vi "Right Click Menu Selected.vi"(8 "error in (no error)":errorcluster, 9 "Panel":string, 10 "Tag":string, 11 "SubPanel User Interface in":refnum<class "SubPanel User Interface.lvclass">) -> (0 "error out":errorcluster, 3 "SubPanel User Interface out":refnum<class "SubPanel User Interface.lvclass">)   [LabVIEW 2020, in "SubPanel User Interface.lvlib" / "SubPanel User Interface.lvclass"]
uses:
  SubPanel User Interface.lvclass
  SubPanel User Interface.lvclass/SubPanel User Interface.ctl
  UI Reference Wrapper/UI Reference Wrapper.lvclass/UI Reference Wrapper.ctl
  UI Reference Wrapper/Read VI Reference.vi
  UI Reference Wrapper/Write VI Reference.vi
  UI Reference Wrapper/UI Reference Wrapper.lvclass
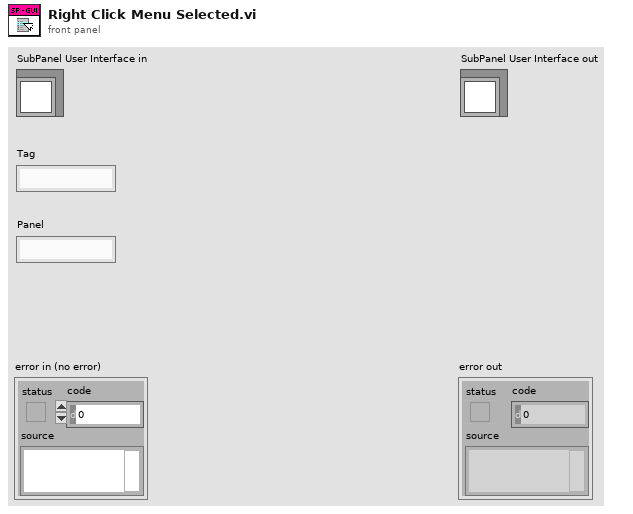
[diagram p1: front panel]
types:
  T1 = enum32{"Invalid", "Standard", "Closed", "Hidden", "Minimized", "Maximized"}
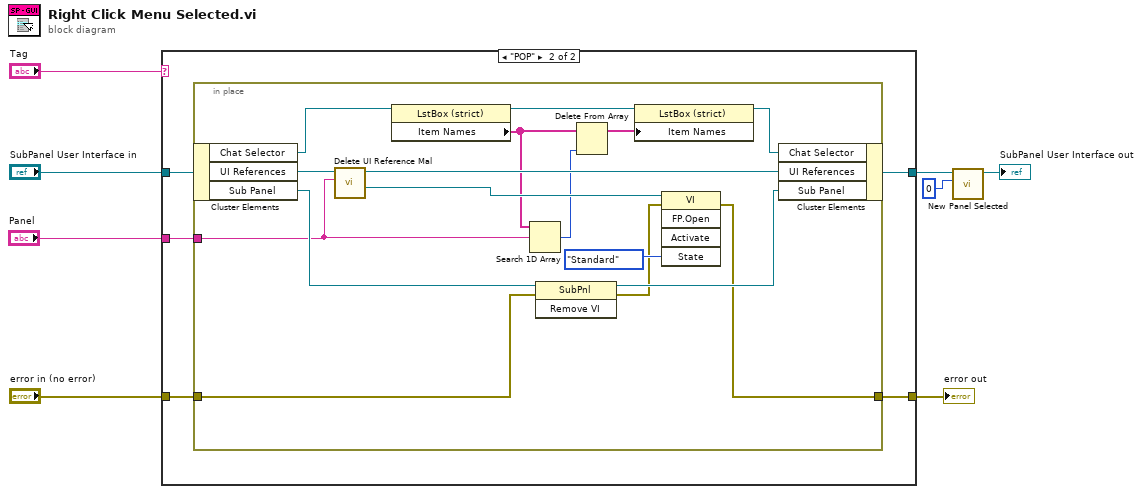
[diagram p0: block diagram]
diagram:
  n1 = case shown="\"POP\"" "Tag" {
    tunnel: "SubPanel User Interface in" -> [w10 w11]
    tunnel: "error in (no error)" -> [w9 w15]
    tunnel: [w10 w14] -> w3
    tunnel: [w9 w12] -> w5
    tunnel: "Panel" -> [_ w13]
    frame "False", Default {
    }
    frame "POP" {
      n2 = in-place {
        in-place-border: w15 -> [w25]
        in-place-border: w13 -> [w23]
        in-place-border: [w24] -> w12
        n3 = in-place-cluster #1(w11) -> ("Chat Selector"=w31:refnum<vi>, "UI References"=w28:refnum<class "UI Reference Wrapper.lvclass">, "Sub Panel"=w26:refnum<vi>)
        n4 = call "Delete UI Reference Mal.vi"("Panel"=w23, "UI Reference Wrapper in"=w28) -> ("VI Refnum"=w22:refnum<vi>, "UI Reference Wrapper out"=w27:refnum<class "UI Reference Wrapper.lvclass">)  [unwired: 6 in, 2 out]
        n5 = property class="LstBox (strict)"(reference=w31) -> (reference out=w20:refnum<vi>, "Item Names"=w17:string[])  [unwired: 1 in, 1 out]
        n6 = Search 1D Array(1D array=w17, element=w23) -> (index of element=w16:i32)  [unwired: 1 in]
        n7 = invoke class="SubPnl" method="Remove VI"(reference=w26, error in=w25) -> (reference out=w29:refnum<vi>, error out=w18:errorcluster)  [unwired: 1 in, 1 out]
        n8 = Delete From Array(array=w17, index=w16) -> (array with subset deleted=w19:string[])  [unwired: 1 in, 1 out]
        n9 = property class="LstBox (strict)"(reference=w20, "Item Names"=w19) -> (reference out=w30:refnum<vi>)  [unwired: 1 in, 1 out]
        n10 = invoke class="VI" method="FP.Open"(reference=w22, error in=w18, "State"=T1."Standard") -> (error out=w24:errorcluster)  [unwired: 2 in, 4 out]
        n11 = in-place-cluster #1("Chat Selector"=w30, "UI References"=w27, "Sub Panel"=w29) -> (w14:refnum<class "SubPanel User Interface.lvclass">)
      }
    }
  }
  "error out" <- w5
  n12 = call "New Panel Selected.vi"("Chat Window"=0, "SubPanel User Interface in"=w3) -> ("SubPanel User Interface out"=→"SubPanel User Interface out":refnum<class "SubPanel User Interface.lvclass">)  [unwired: 8 in, 1 out]
